vi "Dashboard Main.vi"() -> ()   [LabVIEW 2017]
uses:
  <vilib>/Rock Robotics/Network Tables/NT Read Numeric Array.vi
  <vilib>/Rock Robotics/Network Tables/NT Read Boolean.vi
  <vilib>/Rock Robotics/Network Tables/NT Read String.vi
  <vilib>/Rock Robotics/Network Tables/NT Read Number.vi
  <vilib>/Rock Robotics/WPI/Dashboard/WPI_DashboardLogging Global.vi
  <vilib>/Rock Robotics/Network Tables/NT Write Boolean.vi
  <vilib>/Rock Robotics/Network Tables/NT Read String Array.vi
  <vilib>/Rock Robotics/Network Tables/NT Write Number.vi
panel:
  in  "Camera Name":string(combo)="No Camera Selection"
  in  "Camera Settings Right":T1={"Frame Rate"=30, "Compression"=30, "Size"=1, "DB Camera Config"=FALSE} {"Frame Rate" scale=1.0..30.0; "Compression" scale=100.0..-1.0; "Size" items=["640x480", "320x240", "160x120"]}
  in  "Camera Name Right":string(combo)="No Camera Selection"
  out "Camera Info":cluster{"Mbps LED":bool, "Mbps":dbl, "fps":dbl} {"fps" format="%#.1g"; "Mbps" format="%#.1g"}
  in  "Camera Settings":T1={"Frame Rate"=30, "Compression"=30, "Size"=1, "DB Camera Config"=FALSE} {"Frame Rate" scale=1.0..30.0; "Compression" scale=100.0..-1.0; "Size" items=["640x480", "320x240", "160x120"]}
  in  "TCP":refnum<k5>
  in  "Rec Mode":enum32{"Stop", "Record", "Playback"}(radio)
  out "Robot IP":string
  out "Image Message":string="Timeout in Camera Communications"
  in  "Dashboard Tab":T2(tab)
  out "NT Connection":bool
  out "MotorChart R":cluster{"Numeric":dbl, "Numeric":dbl}(graph)
  out "MotorChart L":cluster{"Numeric":dbl, "Numeric":dbl}(graph)
  out "MotorSliders R":cluster{"MotorSlide1":dbl, "MotorSlide2":dbl} {"MotorSlide2" scale=-1.0..1.0 scale format="%#_2e"; "MotorSlide1" scale=-1.0..1.0 scale format="%#_2e"}
  out "MotorSliders L":cluster{"MotorSlide1":dbl, "MotorSlide2":dbl} {"MotorSlide2" scale=-1.0..1.0 scale format="%#_2e"; "MotorSlide1" scale=-1.0..1.0 scale format="%#_2e"}
  out "Gyro":dbl(knob) scale=0.0..360.0
  out "JS1 Z":dbl(slide) scale=-1.0..1.0 scale format="%#_2e"
  out "JS1 Graph":cluster{"X":dbl, "Y":dbl}[](graph)
  out "JS1 Buttons":T3
  out "JS2 Z":dbl(slide) scale=-1.0..1.0 scale format="%#_2e"
  out "JS2 Graph":cluster{"X":dbl, "Y":dbl}[](graph)
  out "JS2 Buttons":T3
  out "Mode":T4(ring)=enum."Auto Disabled"
  in  "Reload Auto Routines":bool
  in  "Starting Position":u16(ring) items=["Any", "Left", "Center", "Right"]
  in  "Run Auto In Teleop":bool
  in  "Right-Right-Right Routine":u16(ring) items=["Auto Line", "Left Scale", "Left Switch", "Right Scale", "Right Switch"]
  in  "Right-Left-Right Routine":u16(ring) items=["Auto Line", "Left Scale", "Left Switch", "Right Scale", "Right Switch"]
  in  "Left-Right-Left Routine":u16(ring) items=["Auto Line", "Left Scale", "Left Switch", "Right Scale", "Right Switch"]
  in  "Left-Left-Left Routine":u16(ring) items=["Auto Line", "Left Scale", "Left Switch", "Right Scale", "Right Switch"]
  out "Arm Control State":string
  out "Auto Control Active":bool
  out "Active Auto Routine":string
  out "Active Start Position":string
  out "Arm Rotate Limit Active":bool
  out "Arm Extend Limit Active":bool
  out "Arm Home Failure":bool
  out "Arm Home Success":bool
  out "Arm":cluster{dbl[], dbl[]}[](graph)
  out "Tree":string(tree)
  out "Camera Image":T5(plugin-control)
  # "HW"
  # "HW"
  # "Joysticks"
  # "Drive Motors"
  # "Front"
  # "Right"
  # "Left"
  # "Back"
  # "Left Start"
  # "Center Start"
  # "Right Start"
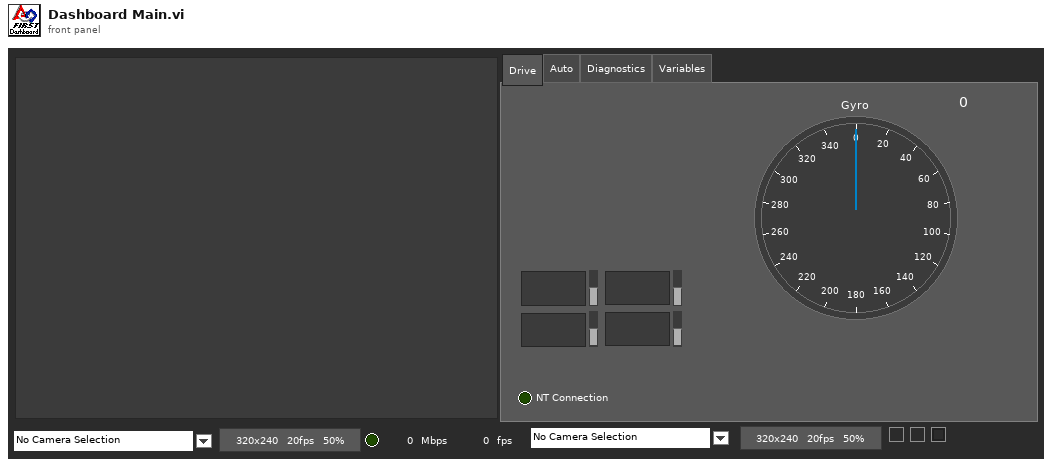
[diagram p1: front panel]
types:
  T1 = cluster{"Frame Rate":i32, "Compression":i32, "Size":u16, "DB Camera Config":bool}
  T2 = enum32{"Drive", "Auto", "Diagnostics", "Variables"}
  T3 = cluster{bool, bool, bool, bool, bool, bool, bool, bool, bool, bool, bool, bool}
  T4 = enum8{"Tele-Op Disabled", "Tele-Op Enabled", "Auto Disabled", "Auto Enabled", "Test Disabled", "Test Enabled", "Disconnected", "No Code", "E-Stop"}
  T5 = typedef "IMAQ Image.ctl" = refnum<image>
  T6 = cluster{"Save Path":path, "Interval (s)":dbl, "Keep":i32}
  T7 = typedef "Image Type" = u32
  T8 = cluster{"IDs":cluster{"RPC field ID":u16, "Unique ID":u16}, "String":string}
  T9 = cluster{"Error Strings":string, "Disable Counts":cluster{u16, u16}, "Rail Faults":cluster{u16, u16, u16}, "Robot IP":string, "DB Mode":u8, "Event Info":cluster{"Name":string, "Type":u8, "Number":u16, "Replay":u8}}
  T10 = cluster{"Storage":cluster{"Disk Free":u64, "RAM Block":u32, "RAM free":u32}, "CPU Utilization":cluster{"CPU % ISR":sgl, "CPU % Time Crit":sgl, "CPU % Timed Str":sgl, "CPU % High":sgl, "CPU % Above":sgl, "CPU % Normal":sgl, "CPU % Low":sgl}, "CAN":cluster{"% Bus Utilization":sgl, "Bus Off Cnt":u32, "TX_FIFO Full Cnt":u32, "Receive Error Cnt":u8, "Transmit Error Cnt":u8}, "HID":cluster{"HID Outputs":u32, "Rumble Low":u16, "Rumble High":u16}[]}
  T11 = cluster{"Status bits":cluster{"Test Mode":bool, "Autonomous":bool, "Enabled":bool, "Code Start":bool, "Brownout":bool, "Reserved 2":bool, "Reserved 3":bool, "E-Stop":bool}, "Code Trace":cluster{"Disabled":bool, "TeleOp":bool, "Auto":bool, "Test":bool}, "Controller Type":enum16{"unknown", "cRIO", "roboRio"}, "Code?":enum16{"unknown", "noCode", "code"}, "Battery V":dbl}
  T12 = cluster{"Control Bits":cluster{"TestMode":bool, "Autonomous":bool, "Enabled":bool, "FMS Present":bool, bool, bool, bool, "E-Stop":bool}, "Team Station ":u8, "Countdown":sgl, "Joystick Values":cluster{"Axes":dbl[], "Buttons":bool[], "POVs":i16[]}[]}
  T13 = cluster{"Axes":dbl[], "Buttons":bool[], "POVs":i16[]}[]
  T14 = cluster{"Axes":dbl[], "Buttons":bool[], "POVs":i16[]}
  T15 = cluster{"Buttons[0]":bool, "Buttons[1]":bool, "Buttons[2]":bool, "Buttons[3]":bool, "Buttons[4]":bool, "Buttons[5]":bool, "Buttons[6]":bool, "Buttons[7]":bool, "Buttons[8]":bool, "Buttons[9]":bool, "Buttons[10]":bool, "Buttons[11]":bool}
  T16 = cluster{"Camera Image":refnum<vi>, "Dashboard Tab":refnum<vi>, "Rec Mode":refnum<vi>, "Tree":refnum<vi>, "Camera Settings":refnum<vi>, "Camera Name":refnum<vi>, "Camera Info":refnum<vi>, "Camera Settings Right":refnum<vi>, "Camera Name Right":refnum<vi>}
  T17 = cluster{"Camera Name Right":string, string, "Saved DB Images Info":cluster{"Save Path":path, "Interval (s)":dbl, "Keep":i32}}
  T18 = cluster{"Camera Name":string, string, "Saved DB Images Info":cluster{"Save Path":path, "Interval (s)":dbl, "Keep":i32}}
  T19 = cluster{"Operation":enum16{"Update", "Clear"}, "Color Box":u32}[]
  T20 = cluster{"Image Size":bool, "Image Type":bool, "Pixel Value":bool, "ROI Information":bool, "Zoom Factor":bool}
  T21 = cluster{"Shift":bool, "Ctrl":bool, "Alt":bool, "Cmd":bool, "Opt":bool}
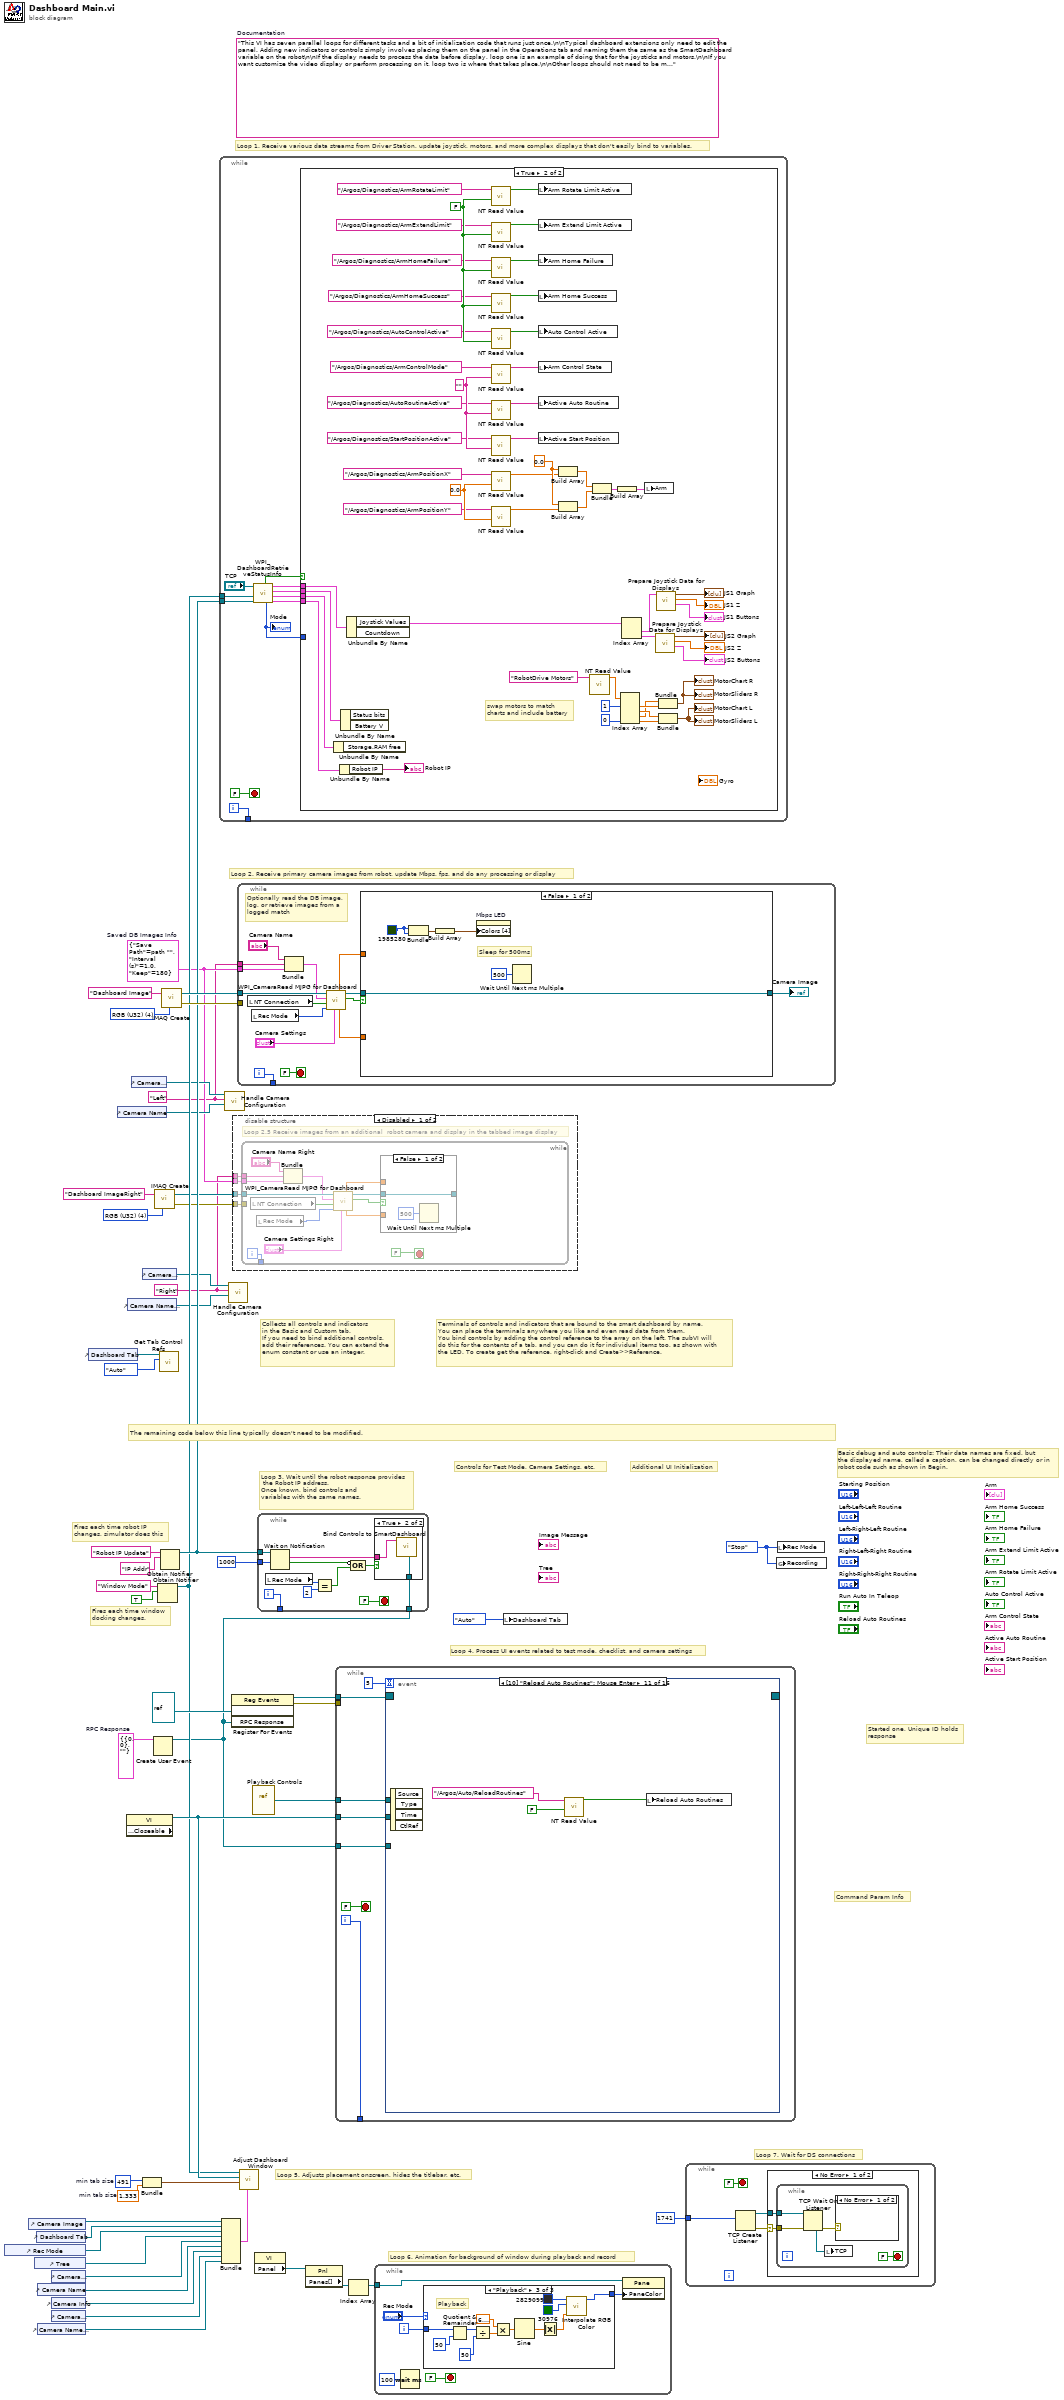
[diagram p0: block diagram]
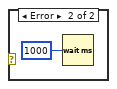
[diagram p5: hidden frame]
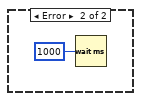
[diagram p6: hidden frame]
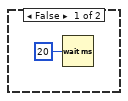
[diagram p7: hidden frame]
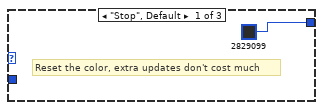
[diagram p8: hidden frame]
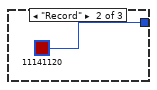
[diagram p9: hidden frame]
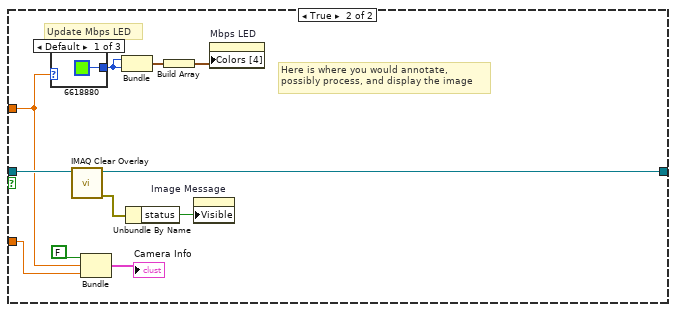
[diagram p10: hidden frame]
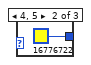
[diagram p11: hidden frame]
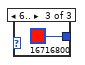
[diagram p12: hidden frame]
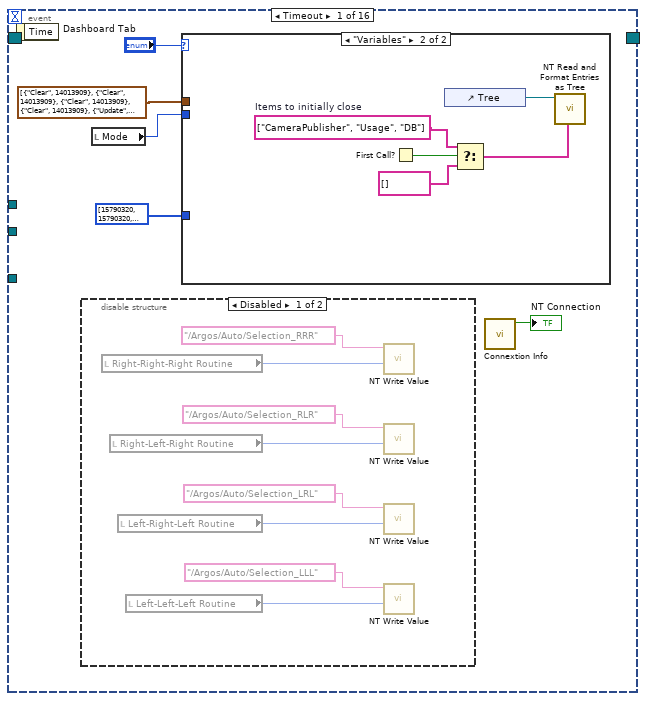
[diagram p13: hidden frame]
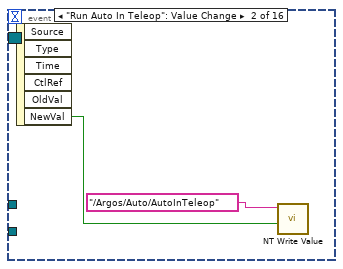
[diagram p16: hidden frame]
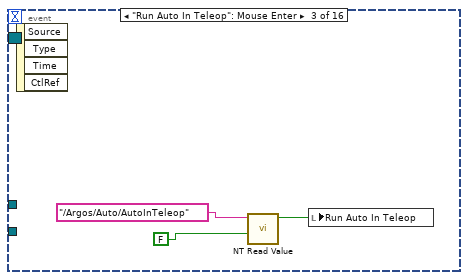
[diagram p17: hidden frame]
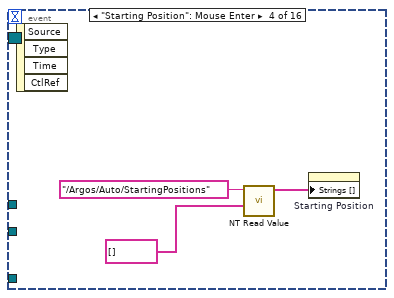
[diagram p18: hidden frame]
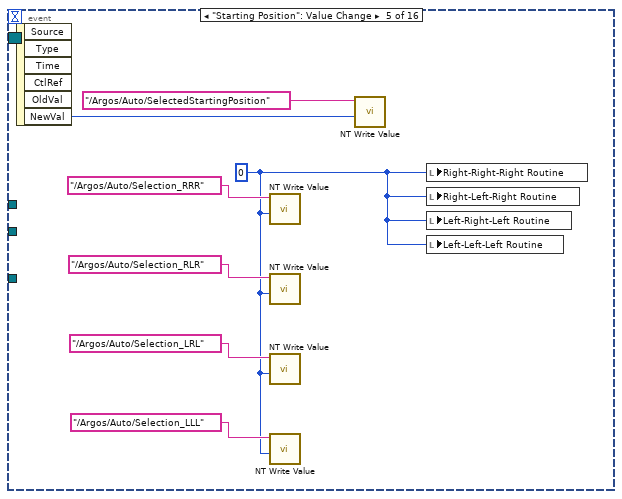
[diagram p19: hidden frame]
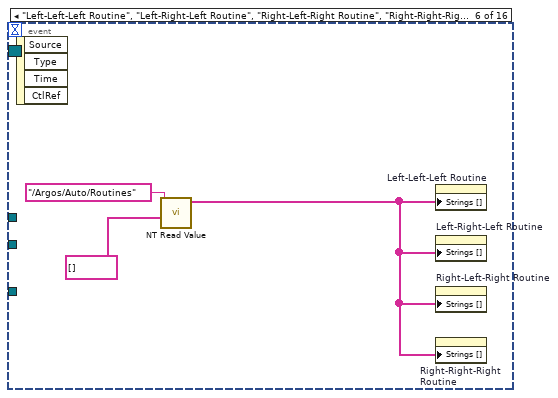
[diagram p20: hidden frame]
diagram:
  w5 = T6 {"Save Path"=path "", "Interval (s)"=1.0, "Keep"=180}  # Saved DB Images Info
  w4 = "Right"
  w3 = "Left"
  w12 = T7 4 items=["Grayscale (U8)", "Grayscale (I16)", "Grayscale (SGL)", "Complex (CSG)", "RGB (U32)", "HSL (U32)", "RGB (U64)"] ("Image Type")
  w20 = T8 {"IDs"={"RPC field ID"=0, "Unique ID"=0}, "String"=""}  # RPC Response
  w30 = 491  # min tab size
  w29 = 1.333  # min tab size
  w35 = enum32{"Stop", "Record", "Playback"}."Stop" ("Rec Mode")
  (unwired) "This VI has seven parallel loops for different tasks and a bit of initialization code that runs just once.\n\nTypical dashboard extensions only need to edit the panel. Adding new indicators or controls simply involves placing them on the panel in the Operations tab and naming them the same as the SmartDashboard variable on the robot\n\nIf the display needs to process the data before display, loop one is an example of doing that for the joysticks and motors.\n\nIf you want customize the video display or perform processing on it, loop two is where that takes place.\n\nOther loops should not need to be modified. They are pretty standard, and document the task they perform."  # Documentation
  w50 = T7 4 items=["Grayscale (U8)", "Grayscale (I16)", "Grayscale (SGL)", "Complex (CSG)", "RGB (U32)", "HSL (U32)", "RGB (U64)"] ("Image Type")
  # "Loop 3. Wait until the robot response provides\n the Robot IP address.\nOnce known, bind controls and\nvariables with the same names."
  # "Command Param Info"
  # "Started one, Unique ID holds\nresponse"
  # "Loop 7. Wait for DS connections"
  # "Basic debug and auto controls: Their data names are fixed, but\nthe displayed name, called a caption, can be changed directly or in\nrobot code such as shown in Begin."
  # "Controls for Test Mode, Camera Settings, etc."
  # "Additional UI Initialization"
  # "Loop 6. Animation for background of window during playback and record"
  # "Fires each time robot IP\nchanges, simulator does this"
  # "Fires each time window\ndocking changes."
  # "Collects all controls and indicators\nin the Basic and Custom tab.\nIf you need to bind additional controls,\nadd their references. You can extend the\nenum constant or use an integer."
  # "The remaining code below this line typically doesn't need to be modified."
  # "Loop 4. Process UI events related to test mode, checklist, and camera settings"
  # "Terminals of controls and indicators that are bound to the smart dashboard by name.\nYou can place the terminals anywhere you like and even read data from them.\nYou bind controls by adding the control reference to the array on the left. The subVI will\ndo this for the contents of a tab, and you can do it for individual items too, as shown with\nthe LED. To create get the reference, right-click and Create>>Reference."
  # "Loop 5. Adjusts placement onscreen, hides the titlebar, etc."
  # "Loop 1. Receive various data streams from Driver Station, update joystick, motors, and more complex displays that don't easily bind to variables."
  # "Loop 2. Receive primary camera images from robot, update Mbps, fps, and do any processing or display"
  n1 = control-ref of="Rec Mode"() -> (w25:refnum<vi>)
  n2 = control-ref of="Camera Image"() -> (w32:refnum<vi>)
  n3 = control-ref of="Tree"() -> (w26:refnum<vi>)
  n4 = control-ref of="Dashboard Tab"() -> (w31:refnum<vi>)
  n5 = control-ref of="Camera Name"() -> (w15:refnum<vi>)
  n6 = control-ref of="Camera Name Right"() -> (w6:refnum<vi>)
  n7 = control-ref of="Camera Settings"() -> (w16:refnum<vi>)
  n8 = control-ref of="Camera Info"() -> (w14:refnum<vi>)
  n9 = control-ref of="Camera Settings Right"() -> (w7:refnum<vi>)
  n10 = control-ref of="Dashboard Tab"() -> (w33:refnum<vi>)
  n11 = control-ref of="Camera Name"() -> (w17:refnum<vi>)
  n12 = property class="VI" props=["Front Panel.Closeable"]() -> (reference out=w34:refnum<vi>)  [unwired: 2 in, 2 out]
  n13 = control-ref of="Camera Name Right"() -> (w8:refnum<vi>)
  n14 = control-ref of="Camera Settings"() -> (w18:refnum<vi>)
  n15 = control-ref of="Camera Settings Right"() -> (w9:refnum<vi>)
  n16 = Bundle("min tab size"=w30, "min tab size"=w29) -> (w28:cluster{"min tab size":i32, "min tab size":dbl})  [unwired: 1 in]
  n17 = Create User Event(user event datatype=w20) -> (user event=w19:refnum<user-event>)  [unwired: 1 in, 1 out]
  n18 = call "IMAQ Create"("Image Name"="Dashboard ImageRight", "Image Type"=w12) -> ("New Image"=w11:T5, "error out"=w10:errorcluster)  [unwired: 2 in, 1 out]
  n19 = Obtain Notifier(name (unnamed)="Window Mode", notification data type=TRUE) -> (notifier out=w23:refnum<notifier>)  [unwired: 2 in, 2 out]
  n20 = call <vilib>:"Get Tab Control Refs.vi"("Page Index"=T2."Auto" ("Dashboard Tab"), "TabControl in"=w33) -> ()  [unwired: 9 in, 1 out]
  n21 = Obtain Notifier(name (unnamed)="Robot IP Update", notification data type="IP Addr" ("name (unnamed)")) -> (notifier out=w24:refnum<notifier>)  [unwired: 2 in, 2 out]
  n22 = call "IMAQ Create"("Image Name"="Dashboard Image", "Image Type"=w50) -> ("New Image"=w48:T5, "error out"=w47:errorcluster)  [unwired: 2 in, 1 out]
  n23 = while {
    tunnel: [w60] -> _
    tunnel: w24 -> [w54]
    tunnel: w23 -> [w51]
    i -> [w60]
    stop <- FALSE stop-if-true
    n24 = call <vilib>:"WPI_DashboardRetrieveStatusInfo.vi"("Binding Refnum"=w54, "Window Mode Notifier"=w51, "TCP Cnx"="TCP") -> ("Power and Errors"=w55:T9, "Robot Metrics"=w58:T10, "Status Info"=w59:T11, "Control Info"=w56:T12, "Robot Mode"=w53:T4, "Process?"=w57:bool)  [unwired: 3 in]
    "Mode" <- w53
    n25 = case shown="True" w57 {
      tunnel: w59 -> [_ w114]
      tunnel: w58 -> [_ w113]
      tunnel: w56 -> [_ w112]
      tunnel: w55 -> [_ w111]
      tunnel: w53 -> [_ _]
      frame False {
        n26 = Wait (ms)(milliseconds to wait=u32 20) -> ()  [unwired: 1 out]
      }
      frame True {
        w68 = 0.0 ("Default Value")
        w73 = 0.0 ("element")
        w79 = "" ("Default Value")
        w90 = FALSE ("Default Value")
        # "swap motors to match\ncharts and include battery"
        n27 = Unbundle By Name(w113) -> ()  [unwired: 1 out]
        n28 = Unbundle By Name(w111) -> ("Robot IP"=→"Robot IP":string)
        n29 = Unbundle By Name(w114) -> ()  [unwired: 2 out]
        n30 = Unbundle By Name(w112) -> ("Joystick Values"=w102:T13)  [unwired: 1 out]
        n31 = call-poly <vilib>:"NT Read Value.vi"("Default Value"=w90, "Name"="/Argos/Diagnostics/ArmRotateLimit") -> ("Boolean"=w89:bool)  [unwired: 8 in, 1 out]
        n32 = call-poly <vilib>:"NT Read Value.vi"("Default Value"=w90, "Name"="/Argos/Diagnostics/ArmExtendLimit") -> ("Boolean"=w88:bool)  [unwired: 8 in, 1 out]
        n33 = call-poly <vilib>:"NT Read Value.vi"("Default Value"=w90, "Name"="/Argos/Diagnostics/ArmHomeFailure") -> ("Boolean"=w87:bool)  [unwired: 8 in, 1 out]
        n34 = call-poly <vilib>:"NT Read Value.vi"("Default Value"=w90, "Name"="/Argos/Diagnostics/ArmHomeSuccess") -> ("Boolean"=w86:bool)  [unwired: 8 in, 1 out]
        n35 = call-poly <vilib>:"NT Read Value.vi"("Default Value"=w90, "Name"="/Argos/Diagnostics/AutoControlActive") -> ("Boolean"=w85:bool)  [unwired: 8 in, 1 out]
        n36 = call-poly <vilib>:"NT Read Value.vi"("Default Value"=w79, "Name"="/Argos/Diagnostics/ArmControlMode") -> ("String"=w78:string)  [unwired: 8 in, 1 out]
        n37 = call-poly <vilib>:"NT Read Value.vi"("Default Value"=w79, "Name"="/Argos/Diagnostics/AutoRoutineActive") -> ("String"=w77:string)  [unwired: 8 in, 1 out]
        n38 = call-poly <vilib>:"NT Read Value.vi"("Default Value"=w79, "Name"="/Argos/Diagnostics/StartPositionActive") -> ("String"=w76:string)  [unwired: 8 in, 1 out]
        n39 = call-poly <vilib>:"NT Read Value.vi"("Default Value"=w68, "Name"="/Argos/Diagnostics/ArmPositionX") -> ("Numeric"=w72:dbl)  [unwired: 8 in, 1 out]
        n40 = call-poly <vilib>:"NT Read Value.vi"("Default Value"=w68, "Name"="/Argos/Diagnostics/ArmPositionY") -> ("Numeric"=w71:dbl)  [unwired: 8 in, 1 out]
        n41 = local write "Arm Rotate Limit Active"(w89) -> ()
        n42 = local write "Arm Extend Limit Active"(w88) -> ()
        n43 = local write "Arm Home Failure"(w87) -> ()
        n44 = local write "Arm Home Success"(w86) -> ()
        n45 = local write "Auto Control Active"(w85) -> ()
        n46 = local write "Arm Control State"(w78) -> ()
        n47 = local write "Active Auto Routine"(w77) -> ()
        n48 = local write "Active Start Position"(w76) -> ()
        n49 = Build Array(w73, w72) -> (w75:dbl[])
        n50 = Build Array(w73, w71) -> (w74:dbl[])
        n51 = call-poly <vilib>:"NT Read Value.vi"("Name"="RobotDrive Motors") -> ("Numeric Array"=w92:dbl[])  [unwired: 9 in, 1 out]
        n52 = Bundle(w75, w74) -> (w70:cluster{dbl[], dbl[]})  [unwired: 1 in]
        n53 = Build Array(w70) -> (w69:cluster{dbl[], dbl[]}[])
        n54 = Index Array(array=w92, index #1=1, index #4=0) -> (element #1=w106:dbl, element #2=w107:dbl, element #3=w105:dbl, element #4=w110:dbl)  [unwired: 2 in]
        n55 = Index Array(array=w102) -> (element #1=w101:T14, element #2=w97:T14)  [unwired: 2 in]
        n56 = local write "Arm"(w69) -> ()
        n57 = call "Prepare Joystick Data for Displays.vi"("Joystick Values"=w97) -> ("Buttons"=→"JS2 Buttons":T15, "Z Axis"=→"JS2 Z":dbl, "Cartesian Data"=→"JS2 Graph":cluster{"X axis":dbl, "X axis":dbl}[])  [unwired: 8 in]
        n58 = call "Prepare Joystick Data for Displays.vi"("Joystick Values"=w101) -> ("Buttons"=→"JS1 Buttons":T15, "Z Axis"=→"JS1 Z":dbl, "Cartesian Data"=→"JS1 Graph":cluster{"X axis":dbl, "X axis":dbl}[])  [unwired: 8 in]
        n59 = Bundle("Numeric"=w105, "Numeric"=w106) -> (→"MotorChart R" →"MotorSliders R":cluster{"Numeric":dbl, "Numeric":dbl})  [unwired: 1 in]
        n60 = Bundle("Numeric"=w107, "Numeric"=w110) -> (→"MotorChart L" →"MotorSliders L":cluster{"Numeric":dbl, "Numeric":dbl})  [unwired: 1 in]
      }
    }
  }
  n61 = Bundle("Camera Image"=w32, "Dashboard Tab"=w31, "Rec Mode"=w25, "Tree"=w26, "Camera Settings"=w16, "Camera Name"=w15, "Camera Info"=w14, "Camera Settings Right"=w7, "Camera Name Right"=w6) -> (w27:T16)  [unwired: 1 in]
  n62 = call "Handle Camera Configuration.vi"("CameraNameRef"=w17, "Display Name"=w3, "ClusterRef"=w18) -> ()  [unwired: 9 in]
  n63 = call "Handle Camera Configuration.vi"("CameraNameRef"=w8, "Display Name"=w4, "ClusterRef"=w9) -> ()  [unwired: 9 in]
  n64 = register-events(refnum<vi> refnum, w19) -> (reference out=w38:refnum<event-registration>, error out=w37:errorcluster)  [unwired: 2 in]
  n65 = disable-structure shown="Disabled" {
    disable-tunnel: w11 -> [w118 _]
    disable-tunnel: w10 -> [w117 _]
    disable-tunnel: w5 -> [w116 _]
    disable-tunnel: w4 -> [w115 _]
    frame Disabled {
      # "Loop 2.5 Receive images from an additional  robot camera and display in the tabbed image display"
      n66 = while {
        tunnel: w118 -> [w132]
        tunnel: w117 -> [_]
        tunnel: [w127] -> _
        tunnel: w116 -> [w122]
        tunnel: w115 -> [w119]
        i -> [w127]
        stop <- FALSE stop-if-true
        n67 = local read "NT Connection"() -> (w123:bool)
        n68 = local read "Rec Mode"() -> (w131:enum32{"Stop", "Record", "Playback"})
        n69 = Bundle("Camera Name Right"="Camera Name Right", w119, "Saved DB Images Info"=w122) -> (w121:T17)  [unwired: 1 in]
        n70 = call <vilib>:"WPI_CameraRead MJPG for Dashboard.vi"("Camera Settings"="Camera Settings Right", "Rec Mode"=w131, "NT Connection"=w123, "Capture Info"=w121, "Refnum in"=w132) -> ("Active"=w126:bool, "Refnum out"=w129:T5, "FPS"=w124:dbl, "Bandwidth (Mbps)"=w125:dbl)  [unwired: 3 in]
        n71 = case shown="False" w126 {
          tunnel: w129 -> [w133 w135]
          tunnel: w125 -> [_ _]
          tunnel: w124 -> [_ _]
          tunnel: [w133 w135] -> _
          frame False {
            n72 = Wait Until Next ms Multiple(millisecond multiple=u32 500) -> ()  [unwired: 1 out]
          }
          frame True {
          }
        }
      }
    }
    frame Enabled {
    }
  }
  n73 = while {
    tunnel: w48 -> [w148]
    tunnel: w47 -> [_]
    tunnel: [w149] -> _
    tunnel: w5 -> [w139]
    tunnel: w3 -> [w136]
    i -> [w149]
    stop <- FALSE stop-if-true
    # "Optionally read the DB image,\nlog, or retrieve images from a\nlogged match"
    n74 = local read "NT Connection"() -> (w140:bool)
    n75 = local read "Rec Mode"() -> (w144:enum32{"Stop", "Record", "Playback"})
    n76 = Bundle("Camera Name"="Camera Name", w136, "Saved DB Images Info"=w139) -> (w138:T18)  [unwired: 1 in]
    n77 = call <vilib>:"WPI_CameraRead MJPG for Dashboard.vi"("Camera Settings"="Camera Settings", "Rec Mode"=w144, "NT Connection"=w140, "Capture Info"=w138, "Refnum in"=w148) -> ("Active"=w146:bool, "Refnum out"=w147:T5, "FPS"=w145:dbl, "Bandwidth (Mbps)"=w143:dbl)  [unwired: 3 in]
    n78 = case shown="False" w146 {
      tunnel: w147 -> [w151 w162]
      tunnel: w143 -> [_ w159]
      tunnel: w145 -> [_ w160]
      tunnel: [w151 w156] -> w141
      frame False {
        w153 = u32 1985280 ("Color Box")
        # "Sleep for 500ms"
        n79 = Bundle("Color Box"=w153, "Color Box"=w153) -> (w154:cluster{"Color Box":u32, "Color Box":u32})  [unwired: 1 out]
        n80 = Build Array(w154) -> (w152:cluster{"Color Box":u32, "Color Box":u32}[])
        n81 = property on="Mbps LED" class="Bool (strict)"("Colors [4]"=w152) -> ()  [unwired: 2 in, 2 out]
        n82 = Wait Until Next ms Multiple(millisecond multiple=u32 500) -> ()  [unwired: 1 out]
      }
      frame True {
        # "Here is where you would annotate,\npossibly process, and display the image"
        # "Update Mbps LED"
        n83 = case shown="Default" w159 {
          tunnel: [u32 6618880 ("Color Box") u32 16776722 ("Color Box") u32 16716800 ("Color Box")] -> w163
          frame Default {
          }
          frame 4, 5 {
          }
          frame 6.. {
          }
        }
        n84 = call "IMAQ Clear Overlay"("Image"=w162) -> ("error out"=w165:errorcluster, "Image Out"=w156:T5)  [unwired: 2 in, 7 out]
        n85 = Bundle(FALSE, "Bandwidth (Mbps)"=w159, "FPS"=w160) -> (→"Camera Info":cluster{bool, "Bandwidth (Mbps)":dbl, "FPS":dbl})  [unwired: 1 in]
        n86 = Bundle("Color Box"=w163, "Color Box"=w163) -> (w164:cluster{"Color Box":u32, "Color Box":u32})  [unwired: 1 out]
        n87 = Unbundle By Name(w165) -> ("status"=w166:bool)
        n88 = Build Array(w164) -> (w161:cluster{"Color Box":u32, "Color Box":u32}[])
        n89 = property on="Image Message" class="Str"("Visible"=w166) -> ()  [unwired: 2 in, 2 out]
        n90 = property on="Mbps LED" class="Bool (strict)"("Colors [4]"=w161) -> ()  [unwired: 2 in, 2 out]
      }
    }
    "Camera Image" <- w141
  }
  n91 = call "Adjust Dashboard Window.vi"("Sizing Refnums"=w27, "Size Constraints"=w28, "VI"=w34, "WIn Mode"=w23) -> ()  [unwired: 8 in]
  n92 = vi-ref "Playback Controls.vi"() -> (w39:refnum<vi>)
  n93 = property class="VI"() -> ("Panel"=w41:refnum<vi>)  [unwired: 2 in, 2 out]
  n94 = while {
    tunnel: w24 -> [w179]
    tunnel: [w177] -> _
    tunnel: u32 1000 ("milliseconds to wait") -> [w176]
    tunnel: w19 -> [w170]
    i -> [w177]
    stop <- FALSE stop-if-true
    n95 = local read "Rec Mode"() -> (w172:enum32{"Stop", "Record", "Playback"})
    n96 = Wait on Notification(notifier=w179, timeout in ms (-1)=w176) -> (notification=w178:string, timed out?=w174:bool)  [unwired: 2 in, 2 out]
    n97 = Equal?(x=w172, y=u16 2 ("Rec Mode")) -> (x = y?=w173:bool)
    n98 = Compound Arithmetic op=OR(invert w174, w173) -> (w175:bool)
    n99 = case shown="True" w175 {
      tunnel: w178 -> [_ w182]
      tunnel: w170 -> [_ w181]
      frame False {
      }
      frame True {
        n100 = call <vilib>:"Bind Controls to SmartDashboard.vi"("RPC ref"=w181, "Server IP Address"=w182) -> ()  [unwired: 10 in]
      }
    }
  }
  n101 = property class="Pnl"(reference=w41) -> ("Panes[]"=w42:refnum<vi>[])  [unwired: 1 in, 2 out]
  n102 = while {
    tunnel: [w187] -> _
    tunnel: w39 -> [w186]
    tunnel: w38 -> [w185]
    tunnel: w37 -> [_]
    tunnel: w34 -> [w184]
    tunnel: w19 -> [w183]
    i -> [w187]
    stop <- FALSE stop-if-true
    n103 = event shown="[10] \"Reload Auto Routines\": Mouse Enter" {
      selector: w185 -> [_ _ _ _ _ _ _ _ _ _ _ _ _ _ _ _]
      dyn-events: [_ _ _ _ _ _ _ _ _ _ _ _ w245 _ _ _] -> _
      timeout: u32 5 ("milliseconds to wait") -> [_ _ _ _ _ _ _ _ _ _ _ _ _ _ _ _]
      tunnel: w186 -> [_ _ _ _ _ _ _ _ _ _ _ _ w247 _ w263 _]
      tunnel: w184 -> [_ _ _ _ _ _ _ _ _ _ _ _ w243 _ _ _]
      tunnel: w183 -> [_ _ _ _ _ _ _ _ _ _ _ _ w241 _ _ _]
      event Timeout {
        n104 = event-data() -> ()  [unwired: 1 in, 1 out]
        n105 = disable-structure shown="Disabled" {
          frame Disabled {
            n106 = local read "Right-Right-Right Routine"() -> (w199:u16)
            n107 = local read "Right-Left-Right Routine"() -> (w200:u16)
            n108 = local read "Left-Right-Left Routine"() -> (w202:u16)
            n109 = local read "Left-Left-Left Routine"() -> (w201:u16)
            n110 = call-poly <vilib>:"NT Write Value.vi"("Numeric"=w199, "Name"="/Argos/Auto/Selection_RRR") -> ()  [unwired: 9 in, 1 out]
            n111 = call-poly <vilib>:"NT Write Value.vi"("Numeric"=w200, "Name"="/Argos/Auto/Selection_RLR") -> ()  [unwired: 9 in, 1 out]
            n112 = call-poly <vilib>:"NT Write Value.vi"("Numeric"=w202, "Name"="/Argos/Auto/Selection_LRL") -> ()  [unwired: 9 in, 1 out]
            n113 = call-poly <vilib>:"NT Write Value.vi"("Numeric"=w201, "Name"="/Argos/Auto/Selection_LLL") -> ()  [unwired: 9 in, 1 out]
          }
          frame Enabled {
          }
        }
        n114 = local read "Mode"() -> (w191:T4)
        n115 = case shown="\"Variables\"" "Dashboard Tab" {
          tunnel: T19 [{"Operation"=enum."Clear", "Color Box"=14013909}, {"Operation"=enum."Clear", "Color Box"=14013909}, {"Operation"=enum."Clear", "Color Box"=14013909}, {"Operation"=enum."Clear", "Color Box"=14013909}, {"Operation"=enum."Update", "Color Box"=14013909}, {"Operation"=enum."Update", "Color Box"=16777215}, {"Operation"=enum."Clear", "Color Box"=14013909}, {"Operation"=enum."Clear", "Color Box"=14013909}, {"Operation"=enum."Clear", "Color Box"=14013909}] -> [_ _]
          tunnel: w191 -> [_ _]
          tunnel: u32[] [15790320, 15790320, 15790320, 15790320, 16777215, 16777215, 15790320, 15790320, 15790320] -> [_ _]
          frame "Diagnostics", Default {
          }
          frame "Variables" {
            w205 = string[] ["CameraPublisher", "Usage", "DB"]  # Items to initially close
            n116 = First Call?() -> (First Call?: T/F=w206:bool)
            n117 = control-ref of="Tree"() -> (w207:refnum<vi>)
            n118 = Select(t=w205, s=w206, f=string[] []) -> (s? t:f=w203:string[])
            n119 = call <vilib>:"NT Read and Format Entries as Tree.vi"("Tags to  Close"=w203, "Tree Refnum"=w207) -> ()  [unwired: 8 in, 2 out]
          }
        }
        n120 = call <vilib>:"Connextion Info.vi"() -> ("Connected"=→"NT Connection":bool)  [unwired: 10 in, 1 out]
      }
      event "Run Auto In Teleop": Value Change {
        n121 = event-data() -> ("NewVal"=w209:bool)  [unwired: 1 in, 5 out]
        n122 = call-poly <vilib>:"NT Write Value.vi"("Boolean"=w209, "Name"="/Argos/Auto/AutoInTeleop") -> ()  [unwired: 9 in, 1 out]
      }
      event "Run Auto In Teleop": Mouse Enter {
        n123 = event-data() -> ()  [unwired: 1 in, 4 out]
        n124 = call-poly <vilib>:"NT Read Value.vi"("Default Value"=FALSE, "Name"="/Argos/Auto/AutoInTeleop") -> ("Boolean"=w210:bool)  [unwired: 8 in, 1 out]
        n125 = local write "Run Auto In Teleop"(w210) -> ()
      }
      event "Starting Position": Mouse Enter {
        n126 = event-data() -> ()  [unwired: 1 in, 4 out]
        n127 = call-poly <vilib>:"NT Read Value.vi"("Default Value"=string[] [], "Name"="/Argos/Auto/StartingPositions") -> ("String Array"=w213:string[])  [unwired: 8 in, 1 out]
        n128 = property on="Starting Position" class="Ring (strict)"("Strings []"=w213) -> ()  [unwired: 2 in, 2 out]
      }
      event "Starting Position": Value Change {
        w216 = u16 0
        n129 = event-data() -> ("NewVal"=w221:u16)  [unwired: 1 in, 5 out]
        n130 = call-poly <vilib>:"NT Write Value.vi"("Numeric"=w216, "Name"="/Argos/Auto/Selection_RRR") -> ()  [unwired: 9 in, 1 out]
        n131 = call-poly <vilib>:"NT Write Value.vi"("Numeric"=w216, "Name"="/Argos/Auto/Selection_RLR") -> ()  [unwired: 9 in, 1 out]
        n132 = call-poly <vilib>:"NT Write Value.vi"("Numeric"=w216, "Name"="/Argos/Auto/Selection_LRL") -> ()  [unwired: 9 in, 1 out]
        n133 = call-poly <vilib>:"NT Write Value.vi"("Numeric"=w216, "Name"="/Argos/Auto/Selection_LLL") -> ()  [unwired: 9 in, 1 out]
        n134 = call-poly <vilib>:"NT Write Value.vi"("Numeric"=w221, "Name"="/Argos/Auto/SelectedStartingPosition") -> ()  [unwired: 9 in, 1 out]
        n135 = local write "Right-Right-Right Routine"(w216) -> ()
        n136 = local write "Right-Left-Right Routine"(w216) -> ()
        n137 = local write "Left-Right-Left Routine"(w216) -> ()
        n138 = local write "Left-Left-Left Routine"(w216) -> ()
      }
      event "Left-Left-Left Routine", "Left-Right-Left Routine", "Right-Left-Right Routine", "Right-Right-Right Routine": Mouse Enter {
        n139 = event-data() -> ()  [unwired: 1 in, 4 out]
        n140 = call-poly <vilib>:"NT Read Value.vi"("Default Value"=string[] [], "Name"="/Argos/Auto/Routines") -> ("String Array"=w223:string[])  [unwired: 8 in, 1 out]
        n141 = property on="Left-Left-Left Routine" class="Ring (strict)"("Strings []"=w223) -> ()  [unwired: 2 in, 2 out]
        n142 = property on="Left-Right-Left Routine" class="Ring (strict)"("Strings []"=w223) -> ()  [unwired: 2 in, 2 out]
        n143 = property on="Right-Left-Right Routine" class="Ring (strict)"("Strings []"=w223) -> ()  [unwired: 2 in, 2 out]
        n144 = property on="Right-Right-Right Routine" class="Ring (strict)"("Strings []"=w223) -> ()  [unwired: 2 in, 2 out]
      }
      event "Left-Left-Left Routine": Value Change {
        n145 = event-data() -> ()  [unwired: 1 in, 6 out]
        n146 = local read "Left-Left-Left Routine"() -> (w227:u16)
        n147 = call-poly <vilib>:"NT Write Value.vi"("Numeric"=w227, "Name"="/Argos/Auto/Selection_LLL") -> ()  [unwired: 9 in, 1 out]
      }
      event "Right-Right-Right Routine": Value Change {
        n148 = event-data() -> ()  [unwired: 1 in, 6 out]
        n149 = local read "Right-Right-Right Routine"() -> (w229:u16)
        n150 = call-poly <vilib>:"NT Write Value.vi"("Numeric"=w229, "Name"="/Argos/Auto/Selection_RRR") -> ()  [unwired: 9 in, 1 out]
      }
      event "Right-Left-Right Routine": Value Change {
        n151 = event-data() -> ()  [unwired: 1 in, 6 out]
        n152 = local read "Right-Left-Right Routine"() -> (w231:u16)
        n153 = call-poly <vilib>:"NT Write Value.vi"("Numeric"=w231, "Name"="/Argos/Auto/Selection_RLR") -> ()  [unwired: 9 in, 1 out]
      }
      event "Left-Right-Left Routine": Value Change {
        n154 = event-data() -> ()  [unwired: 1 in, 6 out]
        n155 = local read "Left-Right-Left Routine"() -> (w233:u16)
        n156 = call-poly <vilib>:"NT Write Value.vi"("Numeric"=w233, "Name"="/Argos/Auto/Selection_LRL") -> ()  [unwired: 9 in, 1 out]
      }
      event "Reload Auto Routines": Mouse Enter {
        n157 = event-data() -> ()  [unwired: 1 in, 4 out]
        n158 = call-poly <vilib>:"NT Read Value.vi"("Default Value"=FALSE, "Name"="/Argos/Auto/ReloadRoutines") -> ("Boolean"=w236:bool)  [unwired: 8 in, 1 out]
        n159 = local write "Reload Auto Routines"(w236) -> ()
      }
      event "Reload Auto Routines": Value Change {
        n160 = event-data() -> ("NewVal"=w237:bool)  [unwired: 1 in, 5 out]
        n161 = call-poly <vilib>:"NT Write Value.vi"("Boolean"=w237, "Name"="/Argos/Auto/ReloadRoutines") -> ()  [unwired: 9 in, 1 out]
      }
      event "Rec Mode": Value Change {
        # "Update globals for recording mode and path to read log from.\nClear when logging and let NetworkTables set path for vision to\nuse."
        n162 = event-data() -> ("NewVal"=w248:enum32{"Stop", "Record", "Playback"})  [unwired: 1 in]
        n163 = global write "WPI_DashboardLogging Global.vi" "Logging Filename"(path "") -> ()
        n164 = global write "WPI_DashboardLogging Global.vi" "Recording"(w248) -> ()
        n165 = case shown="\"Playback\"" w248 {
          tunnel: w247 -> [_ w250 w259]
          tunnel: [_ _ w258] -> w245
          tunnel: [_ _ w257] -> _
          tunnel: w243 -> [_ _ w255]
          tunnel: cluster{i32, i32} {-250, 170} -> [_ _ w254]
          tunnel: [_ _ T20 {"Image Size"=TRUE, "Image Type"=TRUE, "Pixel Value"=TRUE, "ROI Information"=TRUE, "Zoom Factor"=FALSE} ("Image Information Shown:All Elements")] -> w239
          tunnel: [_ _ TRUE ("Zoom Factor")] -> w240
          tunnel: w241 -> [_ _ w251]
          frame Default {
          }
          frame "Stop", "Record" {
            # "Place Window too"
            n166 = invoke class="VI" method="FP.Close"(reference=w250) -> (reference out=w249:refnum<vi>)  [unwired: 2 in, 2 out]
            n167 = invoke class="VI" method="Abort VI"(reference=w249) -> ()  [unwired: 2 in, 3 out]
          }
          frame "Playback" {
            n168 = call "Open Playback Panel.vi"("Offset"=w254, "DB VI Ref"=w255, "Playback in"=w259) -> ("Playback out"=w256:refnum<vi>)  [unwired: 8 in]
            n169 = register-events(w256, w251) -> (reference out=w258:refnum<event-registration>, error out=w257:errorcluster)  [unwired: 2 in]
          }
        }
        n170 = property on="Camera Image" class="ImageControl"("Image Information Shown"=w239, "Image Information Visible"=w240) -> ()  [unwired: 2 in, 2 out]
        n171 = call <vilib>:"WPI_DashboardNT Log FieldName Cache.vi"("Operation"=enum16{"Lookup/Add", "Index", "Clear"}."Clear") -> ()  [unwired: 8 in, 3 out]
      }
      event Panel Close {
        w260 = enum32{"Stop", "Record", "Playback"}."Stop" ("Rec Mode")
        # "Playback window has been closed, abort"
        n172 = event-data() -> ()  [unwired: 1 in, 4 out]
        n173 = local write "Rec Mode"(w260) -> ()
        n174 = global write "WPI_DashboardLogging Global.vi" "Recording"(w260) -> ()
      }
      event Panel Close {
        # "Abort playback window and ourself"
        n175 = event-data() -> ()  [unwired: 1 in, 4 out]
        n176 = invoke class="VI" method="FP.Close"(reference=w263) -> (reference out=w262:refnum<vi>)  [unwired: 2 in, 2 out]
        n177 = invoke class="VI" method="Abort VI"(reference=w262) -> (error out=w261:errorcluster)  [unwired: 2 in, 2 out]
        n178 = invoke class="VI" method="Abort VI"(error in=w261) -> ()  [unwired: 2 in, 3 out]
      }
      event "Tree": Double Click {
        n179 = event-data() -> ("PlatMods"=w269:T21, "Tag"=w266:string)  [unwired: 1 in]
        n180 = Unbundle(w269) -> ("Shift"=w268:bool)  [unwired: 4 out]
        n181 = String Subset(string=w266, length (rest)=1 ("length (rest)")) -> (substring=w265:string)  [unwired: 1 in]
        n182 = Not(x=w268) -> (.not. x?=w267:bool)
        n183 = case shown="\"/\"" w265 {
          tunnel: w266 -> [_ w271]
          tunnel: w267 -> [_ w270]
          frame Default {
          }
          frame "/" {
            n184 = call <vilib>:"NT Update Persistence.vi"("Persistence"=w270, "Name"=w271) -> ()  [unwired: 9 in, 1 out]
          }
        }
      }
    }
  }
  n185 = Index Array(array=w42) -> (element=w40:refnum<vi>)  [unwired: 1 in]
  n186 = while {
    tunnel: w40 -> [w273]
    i -> [w276]
    stop <- FALSE stop-if-true
    n187 = Wait (ms)(milliseconds to wait=u32 100) -> ()  [unwired: 1 out]
    n188 = case shown="\"Playback\"" "Rec Mode" {
      tunnel: w276 -> [_ _ w291]
      tunnel: [u32 2829099 ("Base Color") u32 11141120 ("Target Color") w280] -> w272
      frame "Stop", Default {
        # "Reset the color, extra updates don't cost much"
      }
      frame "Record" {
      }
      frame "Playback" {
        # "Playback"
        n189 = Quotient & Remainder(x=w291, y=u32 50 ("milliseconds to wait")) -> (x-y*floor(x/y)=w287:u32)  [unwired: 1 out]
        n190 = Divide(x=w287, y=u32 50 ("milliseconds to wait")) -> (x/y=w284:dbl)
        n191 = Multiply(x=6.283185307179586, y=w284) -> (x*y=w289:dbl)
        n192 = Sine(x=w289) -> (sin(x)=w288:dbl)
        n193 = Absolute Value(x=w288) -> (abs(x)=w281:dbl)
        n194 = call "Interpolate RGB Color.vi"("Proportion"=w281, "Target Color"=u32 30976, "Base Color"=u32 2829099) -> ("Result Color"=w280:u32)  [unwired: 8 in]
      }
    }
    n195 = property class="Pane"(reference=w273, "PaneColor"=w272) -> ()  [unwired: 1 in, 2 out]
  }
  n196 = local write "Dashboard Tab"(T2."Auto" ("Dashboard Tab")) -> ()
  n197 = while {
    tunnel: u16 1741 ("timeout ms (25000)") -> [w293]
    stop <- FALSE stop-if-true
    n198 = TCP Create Listener(10:w293) -> (0:w292:errorcluster, 3:w294:refnum<k5>)  [unwired: 4 in, 1 out]
    n199 = case shown="No Error" w292 {
      selector: w292 -> [w296 _]
      tunnel: w294 -> [w297 _]
      frame No Error {
        n200 = while {
          tunnel: w297 -> [w300]
          tunnel: w296 -> [w299]
          stop <- FALSE stop-if-true
          n201 = TCP Wait On Listener(8:w299, 11:w300) -> (0:w301:errorcluster, 4:w302:refnum<k5>)  [unwired: 2 in, 3 out]
          n202 = local write "TCP"(w302) -> ()
          n203 = case shown="No Error" w301 {
            frame No Error {
            }
            frame Error {
              n204 = Wait (ms)(milliseconds to wait=u32 1000) -> ()  [unwired: 1 out]
            }
          }
        }
      }
      frame Error {
        n205 = Wait (ms)(milliseconds to wait=u32 1000) -> ()  [unwired: 1 out]
      }
    }
  }
  n206 = global write "WPI_DashboardLogging Global.vi" "Recording"(w35) -> ()
  n207 = local write "Rec Mode"(w35) -> ()
